vi "Skip or Attribute.vi"(11 "Label.Text":string) -> (3 "Checkbox":bool)   [LabVIEW 2019]
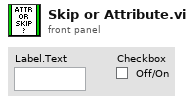
[diagram p1: front panel]
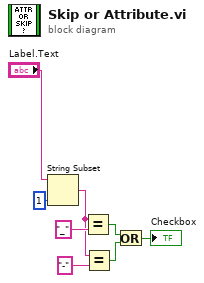
[diagram p0: block diagram]
diagram:
  n1 = String Subset(string="Label.Text", length (rest)=1 ("length (rest)")) -> (substring=w3:string)  [unwired: 1 in]
  n2 = Equal?(x=w3, y="_") -> (x = y?=w6:bool)
  n3 = Equal?(x=w3, y="-") -> (x = y?=w7:bool)
  n4 = Or(x=w6, y=w7) -> (x .or. y?=→"Checkbox":bool)
